vi "Lumen Per Foot To Lux.vi"(9 "Fixture width (in foot)":dbl, 10 "Lumen Per Foot":dbl) -> (2 "Lux":dbl)   [LabVIEW 2016]
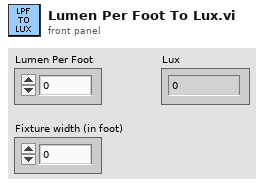
[diagram p1: front panel]
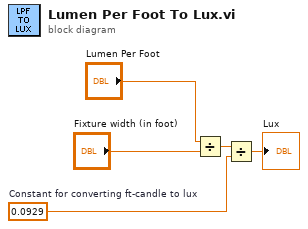
[diagram p0: block diagram]
diagram:
  w1 = 0.0929  # Constant for converting ft-candle to lux
  n1 = Divide(x="Lumen Per Foot", y="Fixture width (in foot)") -> (x/y=w5:dbl)
  n2 = Divide(x=w5, y=w1) -> (x/y=→"Lux":dbl)
